vi "Wiimote Read Accelerometer State.vi"(8 "error in (no error)":errorcluster, 9 "Wiimote Player #":i32=1, 11 "LV WiiMote Interface In":T2) -> (0 "error out":errorcluster, 2 "XYZ Acceleration":T1, 3 "LV WiiMote Interface out":T2)   [LabVIEW 2012, in "LV Wiimote Interface.lvclass"]
uses:
  LV Wiimote Interface.lvclass
  Controls/LV Wiimote Interface.ctl
  Controls/XYZ Acceleration.ctl
  C:/Program Files/National Instruments/LabVIEW 2012/vi.lib/LabVIEW Hacker/WiiMote/Dependencies/WiimoteLib.dll
  Program Files/National Instruments/LabVIEW 2012/vi.lib/LabVIEW Hacker/WiiMote/Dependencies/WiimoteLib.dll
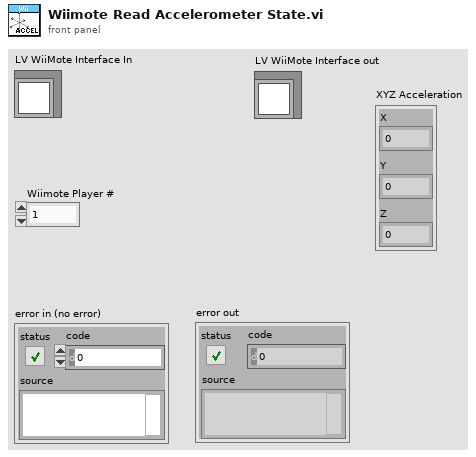
[diagram p1: front panel]
types:
  T1 = typedef "LV Wiimote Interface.lvclass/XYZ Acceleration.ctl" = cluster{"X":sgl, "Y":sgl, "Z":sgl}
  T2 = typedef "LV Wiimote Interface.ctl" = refnum<class "LV Wiimote Interface.lvclass">
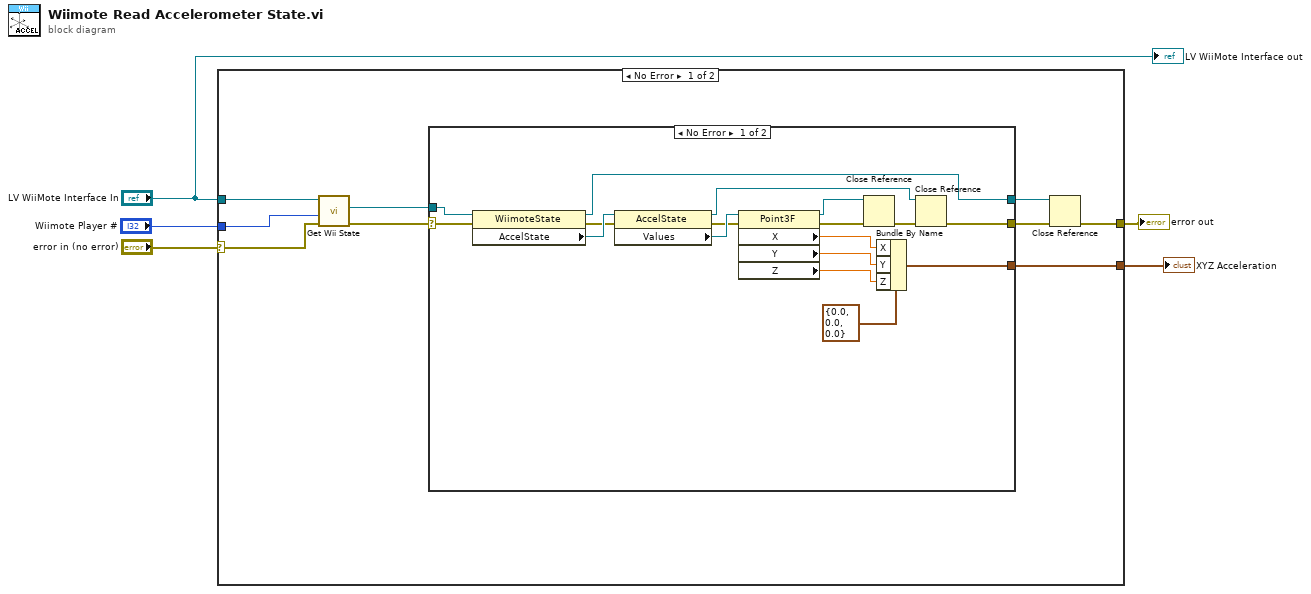
[diagram p0: block diagram]
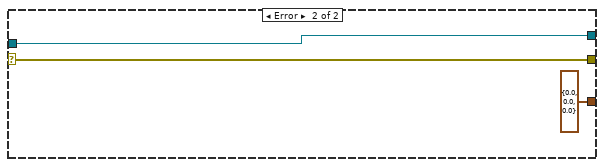
[diagram p2: hidden frame]
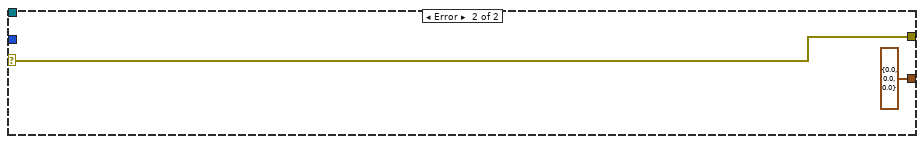
[diagram p3: hidden frame]
diagram:
  n1 = case shown="No Error" "error in (no error)" {
    selector: "error in (no error)" -> [w13 w36]
    tunnel: "LV WiiMote Interface In" -> [w14 _]
    tunnel: "Wiimote Player #" -> [w7 _]
    tunnel: [w10 w36] -> w2
    tunnel: [w8 T1 {"X"=0.0, "Y"=0.0, "Z"=0.0} ("XYZ Acceleration")] -> w1
    frame No Error {
      n2 = call "Get Wii State.vi"("error in (no error)"=w13, "Wiimote Player #"=w7, "LV Wiimote Interface in"=w14) -> ("error out"=w12:errorcluster, "WiimoteState"=w6:refnum<k24>)  [unwired: 6 in, 1 out]
      n3 = case shown="No Error" w12 {
        selector: w12 -> [w29 w34]
        tunnel: w6 -> [w31 w33]
        tunnel: [w20 w34] -> w11
        tunnel: [w21 w33] -> w9
        tunnel: [w15 T1 {"X"=0.0, "Y"=0.0, "Z"=0.0} ("XYZ Acceleration")] -> w8
        frame No Error {
          n4 = property class="WiimoteState"(reference=w31, error in=w29) -> (reference out=w21:refnum<k24>, error out=w27:errorcluster, "AccelState"=w28:refnum<k24>)
          n5 = property class="AccelState"(reference=w28, error in=w27) -> (reference out=w22:refnum<k24>, error out=w24:errorcluster, "Values"=w25:refnum<k24>)
          n6 = property class="Point3F"(reference=w25, error in=w24) -> (reference out=w23:refnum<k24>, error out=w26:errorcluster, "X"=w18:sgl, "Y"=w17:sgl, "Z"=w16:sgl)
          n7 = Close Reference(reference=w23, error in (no error)=w26) -> (error out=w30:errorcluster)
          n8 = Bundle By Name(cluster=T1 {"X"=0.0, "Y"=0.0, "Z"=0.0} ("XYZ Acceleration"), "X"=w18, "Y"=w17, "Z"=w16) -> (w15:T1)
          n9 = Close Reference(reference=w22, error in (no error)=w30) -> (error out=w20:errorcluster)
        }
        frame Error {
        }
      }
      n10 = Close Reference(reference=w9, error in (no error)=w11) -> (error out=w10:errorcluster)
    }
    frame Error {
    }
  }
  "error out" <- w2
  "XYZ Acceleration" <- w1
  "LV WiiMote Interface out" <- "LV WiiMote Interface In"
